vi "MathCad Open.vi"(8 "error in (no error)":errorcluster, 10 "Visible":bool=TRUE, 11 "File Path":T2) -> (0 "error out (no error)":errorcluster, 3 "Mathcad Reference":T1)   [LabVIEW 2015]
doc: "Opens a Mathcad Worksheet (*.mcd) specified by \"File Path\" using the ActiveX Automation Interface. Also, opens ActiveX References to the Worksheet, Worksheets, and Application Class.\n\nInputs\nFile Path - File path to *.mcd file to Open. If an invalid file path is specified, Mathcad will still Open with no worksheets open. The Application ActiveX Reference can still be used.\n\nOutputs\nMathcad Reference (Cluster- 3 Elements)\n Mathcad Application-Reference to the IMathcadApplication Class\n Worksheets Reference-Reference to the Worksheets Class that contains the Worksheet (*.mcd file) that was opened\n Worksheet Reference- Reference to the Worksheet Class that was opened to the file."
uses:
  File Path Open Mathcad.ctl
  Mathcad Reference.ctl
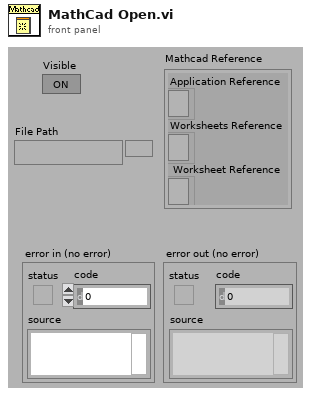
[diagram p1: front panel]
types:
  T1 = typedef "Mathcad Reference.ctl" = cluster{"Application Reference":refnum<k7>, "Worksheets Reference":refnum<k7>, " Worksheet Reference":refnum<k7>}
  T2 = typedef "File Path Open Mathcad.ctl" = path
  T3 = cluster{"Application Reference ":refnum<k7>, "Worksheets Reference":refnum<k7>, "Worksheet Reference":refnum<k7>}
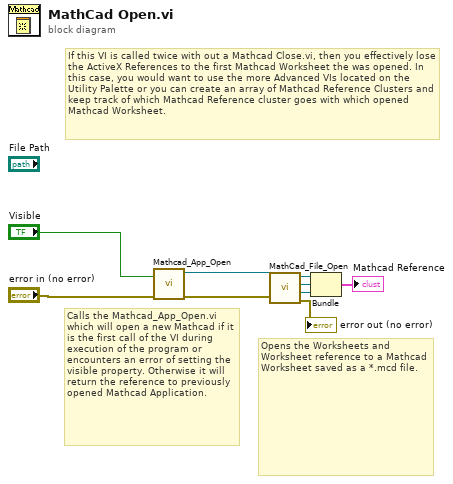
[diagram p0: block diagram]
diagram:
  # "If this VI is called twice with out a Mathcad Close.vi, then you effectively lose the ActiveX References to the first Mathcad Worksheet the was opened. In this case, you would want to use the more Advanced VIs located on the Utility Palette or you can create an array of Mathcad Reference Clusters and keep track of which Mathcad Reference cluster goes with which opened Mathcad Worksheet."
  # "Opens the Worksheets and Worksheet reference to a Mathcad Worksheet saved as a *.mcd file."
  # "Calls the Mathcad_App_Open.vi which will open a new Mathcad if it is the first call of the VI during execution of the program or encounters an error of setting the visible property. Otherwise it will return the reference to previously opened Mathcad Application."
  n1 = call "Mathcad_App_Open.vi"("Visible"="Visible", "error in (no error)"="error in (no error)") -> ("error out (no error)"=w1:errorcluster, "Mathcad.IMathcadApplication"=w5:refnum<k7>)  [unwired: 8 in]
  n2 = call "MathCad_File_Open.vi"("error in (no error)"=w1, "Mathcad.IMathcadApplication"=w5) -> ("error out (no error)"=→"error out (no error)":errorcluster, "Worksheet Reference"=w2:refnum<k7>, "Worksheets Reference"=w3:refnum<k7>, "Application Reference"=w4:refnum<k7>)  [unwired: 6 in]
  n3 = Bundle("Application Reference"=w4, "Worksheets Reference"=w3, "Worksheet Reference"=w2) -> (→"Mathcad Reference":T3)  [unwired: 1 in]
